vi "GetNextCommand.vi"(8 "error in (no error)":errorcluster, 11 "PathTokenizer in":refnum<class "PathTokenizer.lvclass">) -> (0 "error out":errorcluster, 1 "Index":i32, 2 "Character":string, 3 "PathTokenizer out":refnum<class "PathTokenizer.lvclass">, 4 "Found?":bool)   [LabVIEW 2020, in "PathTokenizer.lvclass"]
uses:
  PathTokenizer.lvclass
  PathTokenizer.lvclass/PathTokenizer.ctl
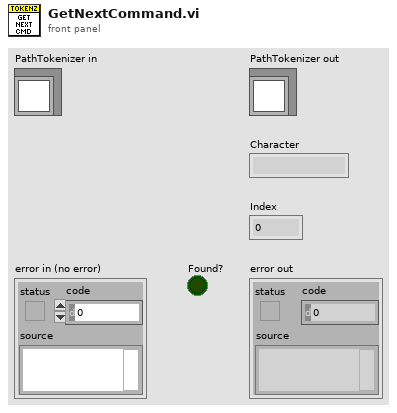
[diagram p1: front panel]
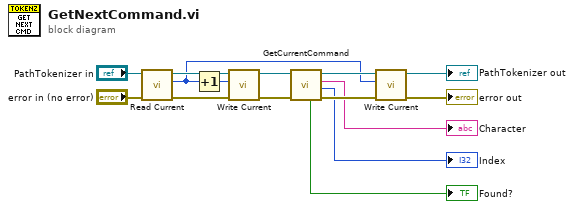
[diagram p0: block diagram]
diagram:
  n1 = call "Read Current.vi"("error in (no error)"="error in (no error)", "PathTokenizer in"="PathTokenizer in") -> ("error out"=w14:errorcluster, "Current"=w1:i32, "PathTokenizer out"=w15:refnum<class "PathTokenizer.lvclass">)  [unwired: 7 in]
  n2 = Increment(x=w1) -> (x+1=w5:i32)
  n3 = call "Write Current.vi"("error in (no error)"=w14, "Current"=w5, "PathTokenizer in"=w15) -> ("error out"=w12:errorcluster, "PathTokenizer out"=w13:refnum<class "PathTokenizer.lvclass">)  [unwired: 7 in]
  n4 = call "GetCurrentCommand.vi"("error in (no error)"=w12, "PathTokenizer in"=w13) -> ("error out"=w10:errorcluster, "Index"=→"Index":i32, "Character"=→"Character":string, "PathTokenizer out"=w11:refnum<class "PathTokenizer.lvclass">, "Found?"=→"Found?":bool)  [unwired: 5 in]
  n5 = call "Write Current.vi"("error in (no error)"=w10, "Current"=w1, "PathTokenizer in"=w11) -> ("error out"=→"error out":errorcluster, "PathTokenizer out"=→"PathTokenizer out":refnum<class "PathTokenizer.lvclass">)  [unwired: 7 in]
